vi "sv_Convert Elapsed Time to Counter Rollover Ticks.vi"(9 "counter maximum value":u64=4294967296, 10 "counter timebase (Hz)":dbl=13107200.0 format="%#_10f", 11 "elapsed time (s)":dbl) -> (1 "rollovers":u64, 2 "elapsed rollover ticks":u64, 3 "elapsed ticks":u64)   [LabVIEW 2017]
doc: "Converts elapsed time to ticks using the counter timebase to convert seconds to ticks. For a given counter maximum value, this function also returns the number of counter rollovers and the number of ticks associated with those rollovers."
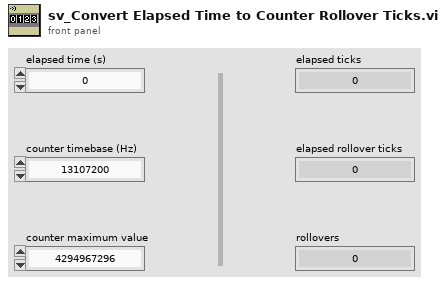
[diagram p1: front panel]
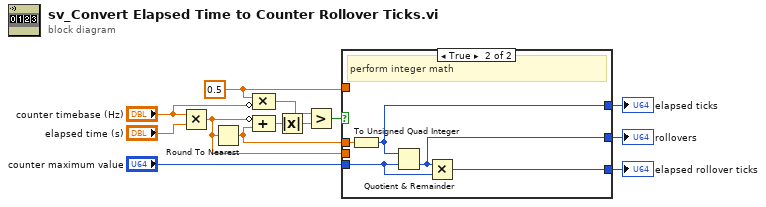
[diagram p0: block diagram]
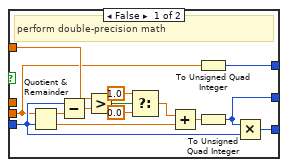
[diagram p2: hidden frame]
diagram:
  w6 = 0.5 ("value")
  n1 = Multiply(x="counter timebase (Hz)", y="elapsed time (s)") -> (x*y=w7:dbl)
  n2 = Round To Nearest(number=w7) -> (nearest integer value=w8:dbl)
  n3 = Compound Arithmetic op=MULTIPLY(w6, invert "counter timebase (Hz)") -> (w10:dbl)
  n4 = Compound Arithmetic op=ADD(invert w7, w8) -> (w12:dbl)
  n5 = Absolute Value(x=w12) -> (abs(x)=w9:dbl)
  n6 = Greater?(x=w10, y=w9) -> (0:w3:bool)
  n7 = case shown="True" w3 {
    tunnel: w8 -> [_ w32]
    tunnel: "counter maximum value" -> [w27 w31]
    tunnel: w7 -> [w15 _]
    tunnel: w6 -> [w24 _]
    tunnel: [w17 w30] -> w5
    tunnel: [w16 w29] -> w4
    tunnel: [w14 w28] -> w2
    frame False {
      # "perform double-precision math"
      n8 = Quotient & Remainder(x=w15, y=w27) -> (x-y*floor(x/y)=w26:dbl, floor(x/y)=w19:dbl)
      n9 = Subtract(x=w27, y=w26) -> (x-y=w25:dbl)
      n10 = Greater?(x=w24, y=w25) -> (0:w23:bool)
      n11 = Select(t=1.0, s=w23, f=0.0) -> (s? t:f=w20:dbl)
      n12 = Add(x=w20, y=w19) -> (x+y=w18:dbl)
      n13 = To Unsigned Quad Integer(1:w15) -> (0:w14:u64)
      n14 = To Unsigned Quad Integer(1:w18) -> (0:w16:u64)
      n15 = Multiply(x=w16, y=w27) -> (x*y=w17:u64)
    }
    frame True {
      # "perform integer math"
      n16 = To Unsigned Quad Integer(1:w32) -> (0:w28:u64)
      n17 = Quotient & Remainder(x=w28, y=w31) -> (floor(x/y)=w29:u64)  [unwired: 1 out]
      n18 = Multiply(x=w29, y=w31) -> (x*y=w30:u64)
    }
  }
  "elapsed rollover ticks" <- w5
  "rollovers" <- w4
  "elapsed ticks" <- w2
